vi "Save PartsMeasurementMapping to DB.vi"(8 "error in":errorcluster, 10 "GTron DB":path=path "D:/SQL Database/Gtron Database.db", 11 "output cluster":T1) -> (0 "error out":errorcluster)   [LabVIEW 2019, in "DataLogger.lvclass"]
uses:
  DataLogger.lvclass
  <vilib>/drjdpowell/SQLite Library/SQL Statement/SQL Statement.lvclass
  <vilib>/drjdpowell/SQLite Library/SQL Connection/Connection.lvclass
  <vilib>/drjdpowell/SQLite Library/SQL Connection/Open (path).vi
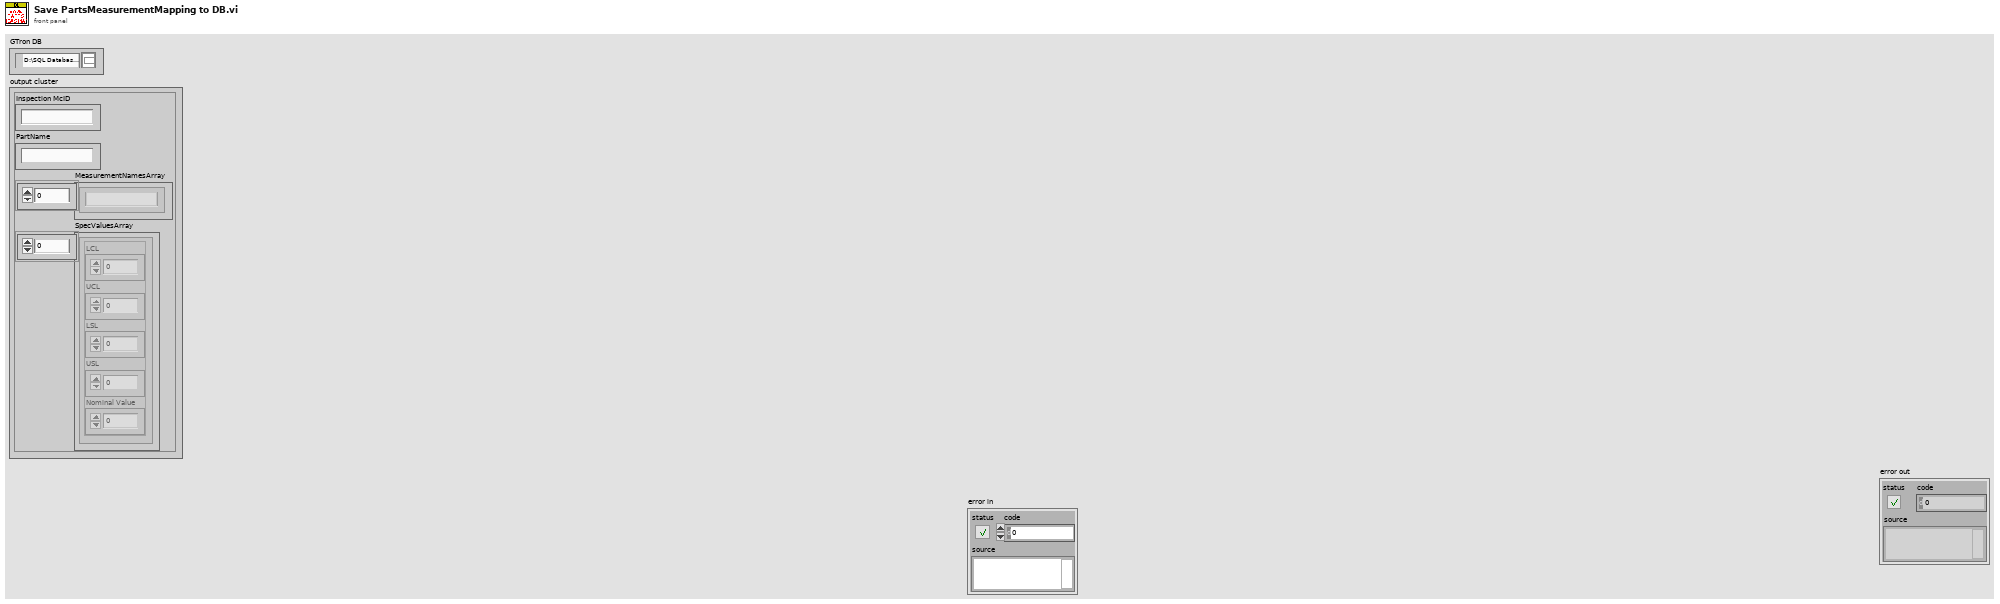
[diagram p1: front panel]
types:
  T1 = cluster{"Inspection McID":string, "PartName":string, "MeasurementNamesArray":string[], "SpecValuesArray":cluster{"LCL":dbl, "UCL":dbl, "LSL":dbl, "USL":dbl, "Nominal Value":dbl}[]}
  T2 = cluster{"LCL":dbl, "UCL":dbl, "LSL":dbl, "USL":dbl, "Nominal Value":dbl}[]
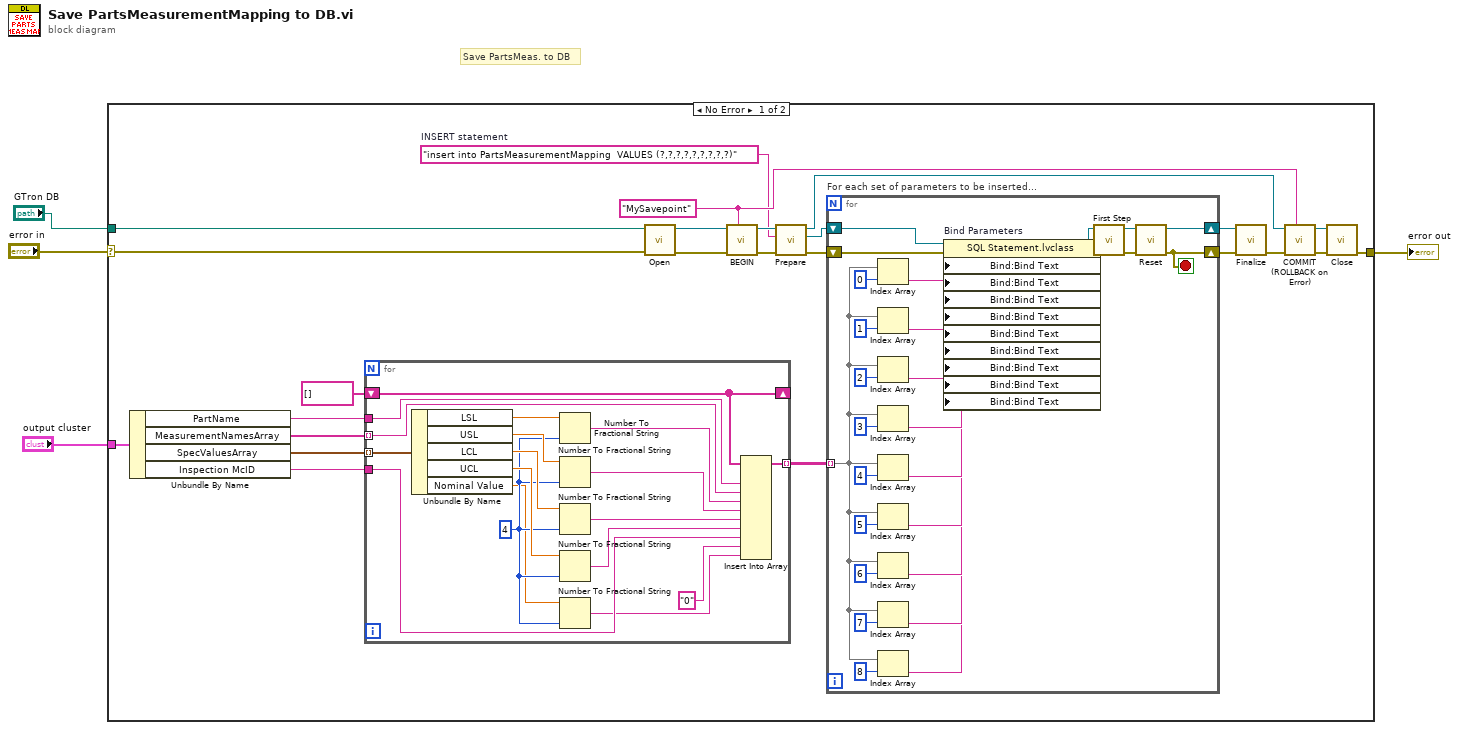
[diagram p0: block diagram]
diagram:
  # "Save PartsMeas. to DB"
  n1 = case shown="No Error" "error in" {
    selector: "error in" -> [w6 w74]
    tunnel: [w14 w74] -> w4
    tunnel: "output cluster" -> [w12 _]
    tunnel: "GTron DB" -> [w5 _]
    frame No Error {
      w26 = "MySavepoint" ("Savepoint name")
      w13 = "insert into PartsMeasurementMapping  VALUES (?,?,?,?,?,?,?,?,?)"  # INSERT statement
      n2 = Unbundle By Name(w12) -> ("PartName"=w11:string, "MeasurementNamesArray"=w10:string[], "SpecValuesArray"=w9:T2, "Inspection McID"=w7:string)
      n3 = for {
        shift-right: [w46] -> _
        shift-left: string[] [] -> [w46]
        tunnel: w11 -> [w45]
        tunnel: w10 -> [w44] mode=indexing
        tunnel: w9 -> [w43] mode=indexing
        tunnel: [w34] -> w17 mode=indexing
        tunnel: w7 -> [w33]
        w32 = i16 4 ("precision (6)")
        n4 = Unbundle By Name(w43) -> ("LSL"=w42:dbl, "USL"=w41:dbl, "LCL"=w40:dbl, "UCL"=w39:dbl, "Nominal Value"=w31:dbl)
        n5 = Number To Fractional String(number=w42, precision (6)=w32) -> (F-format string=w38:string)  [unwired: 2 in]
        n6 = Number To Fractional String(number=w41, precision (6)=w32) -> (F-format string=w37:string)  [unwired: 2 in]
        n7 = Number To Fractional String(number=w40, precision (6)=w32) -> (F-format string=w36:string)  [unwired: 2 in]
        n8 = Number To Fractional String(number=w39, precision (6)=w32) -> (F-format string=w35:string)  [unwired: 2 in]
        n9 = Number To Fractional String(number=w31, precision (6)=w32) -> (F-format string=w29:string)  [unwired: 2 in]
        n10 = Insert Into Array(array=w46, new element #1=w45, new element #2=w44, new element #3=w38, new element #4=w37, new element #5=w36, new element #6=w35, new element #7=w33, new element #8="0" ("new element/subarray"), new element #9=w29) -> (w34:string[])  [unwired: 1 in]
      }
      n11 = call-poly <vilib>:"Open.vi"("error in (no error)"=w6, "db file"=w5) -> ("error out"=w18:errorcluster, "SQLite Connection"=w19:refnum<class "Connection.lvclass">)  [unwired: 8 in]
      n12 = call <vilib>:"BEGIN.vi"("Savepoint name"=w26, "error in (no error)"=w18, "Connection in"=w19) -> ("error out"=w25:errorcluster, "Connection out"=w24:refnum<class "Connection.lvclass">)  [unwired: 7 in]
      n13 = call <vilib>:"Prepare.vi"("error in (no error)"=w25, "SQL"=w13, "SQLite Connection in"=w24) -> ("error out"=w21:errorcluster, "SQL Statement"=w20:refnum<class "SQL Statement.lvclass">, "SQLite Connection"=w27:refnum<class "Connection.lvclass">)  [unwired: 4 in, 2 out]
      n14 = for "For each set of parameters to be inserted..." {
        shift-right: [w71] -> w22
        shift-left: w20 -> [w73]
        shift-right: [w70] -> w23
        shift-left: w21 -> [w72]
        tunnel: w17 -> [w53] mode=indexing
        stop <- w70 stop-if-true
        n15 = Index Array(array=w53, index=0) -> (element=w59:string)
        n16 = Index Array(array=w53, index=1) -> (element=w58:string)
        n17 = Index Array(array=w53, index=2) -> (element=w57:string)
        n18 = Index Array(array=w53, index=3) -> (element=w56:string)
        n19 = Index Array(array=w53, index=4) -> (element=w55:string)
        n20 = Index Array(array=w53, index=5) -> (element=w54:string)
        n21 = Index Array(array=w53, index=6) -> (element=w49:string)
        n22 = Index Array(array=w53, index=7) -> (element=w48:string)
        n23 = Index Array(array=w53, index=8) -> (element=w47:string)
        n24 = property on="Bind Parameters" class="SQL Statement.lvclass"(reference=w73, error in=w72, "Bind:Bind Text"=w59, "Bind:Bind Text"=w58, "Bind:Bind Text"=w57, "Bind:Bind Text"=w56, "Bind:Bind Text"=w55, "Bind:Bind Text"=w54, "Bind:Bind Text"=w49, "Bind:Bind Text"=w48, "Bind:Bind Text"=w47) -> (reference out=w69:refnum<class "SQL Statement.lvclass">, error out=w68:errorcluster)
        n25 = call <vilib>:"First Step.vi"("error in (no error)"=w68, "SQL Statement in"=w69) -> ("error out"=w67:errorcluster, "SQL Statement"=w66:refnum<class "SQL Statement.lvclass">)  [unwired: 7 in, 1 out]
        n26 = call <vilib>:"Reset.vi"("error in (no error)"=w67, "SQL Statement in"=w66) -> ("error out"=w70:errorcluster, "SQL Statement"=w71:refnum<class "SQL Statement.lvclass">)  [unwired: 8 in]
      }
      n27 = call <vilib>:"Finalize.vi"("error in (no error)"=w23, "SQL Statement in"=w22) -> ("error out"=w28:errorcluster)  [unwired: 9 in]
      n28 = call <vilib>:"COMMIT (ROLLBACK on Error).vi"("Savepoint name"=w26, "error in (no error)"=w28, "Connection in"=w27) -> ("error out"=w15:errorcluster, "Connection out"=w16:refnum<class "Connection.lvclass">)  [unwired: 7 in]
      n29 = call-dynamic "Close.vi"("error in (no error)"=w15, "SQLite Connection in"=w16) -> ("error out"=w14:errorcluster)  [unwired: 9 in]
    }
    frame Error {
    }
  }
  "error out" <- w4
